vi "TEST-SAOMM-Externaloffset.vi"(0 "Hexapod VRN":refnum<visa-resource-name>="COM4", 1 "Active Refnum":refnum<vi>, 2 "PrAMS-ACK":refnum<vi>, 7 "output cluster":T2, 12 "offset_cluster":T1, 13 "MessageType":cluster{string[], u32[]}={["emtError", "emtAreYouThere", "emtAcknowledgment", "emtGetClientType", "emtClientType", "emtGetImageExposureTime", "emtSetImageExposureTime", "emtImageExposureTime", "emtGetOptimalExposureTime", "emtSetOptimalExposureTime", "emtOptimalExposureTime", "emtGetImageEMGain", "emtSetImageEMGain", "emtImageEMGain", "emtGetFPGACtrl", "emtSetFPGACtrl", "emtFPGACtrl", "emtGetImageWidth", "emtSetImageWidth", "emtImageWidth", "emtGetImageHeight", "emtSetImageHeight", "emtImageHeight", "emtGetImageBinning", "emtSetImageBinning", "emtImageBinning", "emtGetImageDisplayFrameRate", "emtSetImageDisplayFrameRate", "emtImageDisplayFrameRate", "emtGetROIWidth", "emtSetROIWidth", "emtROIWidth", "emtGetROIHeight", "emtSetROIHeight", "emtROIHeight", "emtGetROIXOffset", "emtSetROIXOffset", "emtROIXOffset", "emtGetROIYOffset", "emtSetROIYOffset", "emtROIYOffset", "emtStartAcquisition", "mtStopAcquisition", "emtAcquisitionStarted", "emtAcquisitionStopped", "emtGetFalconImage", "emtFalconImage"], [1, 2, 3, 4, 5, 1001, 1101, 1201, 1002, 1102, 1202, 1003, 1103, 1203, 1004, 1104, 1204, 1005, 1105, 1205, 1006, 1106, 1206, 1007, 1107, 1207, 1008, 1108, 1208, 1009, 1109, 1209, 1010, 1110, 1210, 1011, 1111, 1211, 1012, 1112, 1212, 1130, 1131, 1150, 1151, 1070, 1270]}) -> (8 "Error":bool)   [LabVIEW 2019]
uses:
  Polymorphics/Num2littleEndian(DBL).vi
panel:
  out "First Run":bool
  in  "IncUV":dbl caption="Incrément" format="%.4g"
  in  "IncXYZ":dbl caption="Incrément" format="%.3f"
  in  "V+":bool
  in  "V-":bool
  in  "U+":bool
  in  "U-":bool
  in  "Z+":bool
  in  "Z-":bool
  in  "Y+":bool
  in  "Y-":bool
  in  "X+":bool
  in  "X-":bool
  in  "keep-active":bool caption="Laisser ouvert ?"
  in  "Signature":u32=1886544237
  in  "Cancel":bool
  in  "Send":bool
  in  "X":dbl caption="Pos" min=-5.0 max=5.0 format="%.4f"
  in  "Y":dbl caption="Pos" min=-5.0 max=5.0 format="%.4f"
  in  "Z":dbl caption="Pos" min=-5.0 max=5.0 format="%.4f"
  in  "U":dbl caption="Pos" min=-1.0 max=1.0 format="%.4f"
  in  "V":dbl caption="Pos" min=-1.0 max=1.0 format="%.4f"
  # "DÉPLACEMENTS"
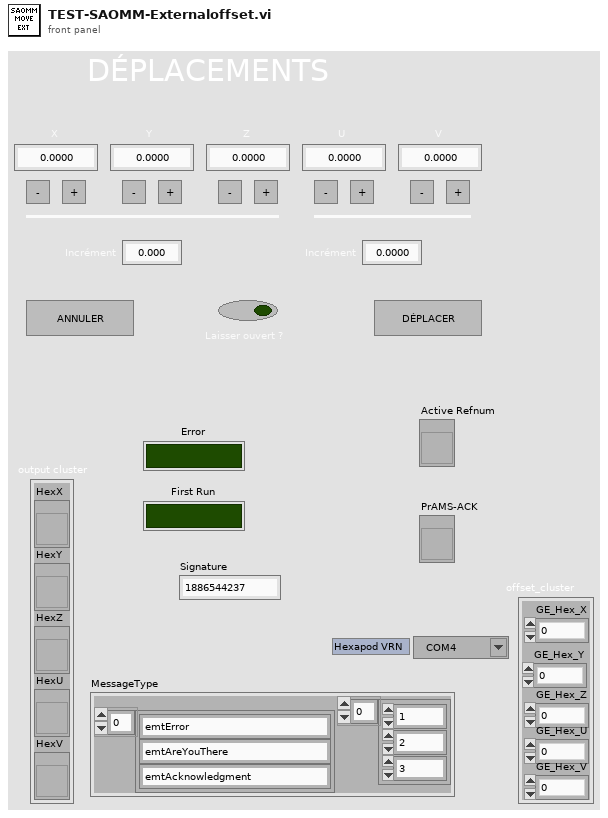
[diagram p1: front panel]
types:
  T1 = cluster{"GE_Hex_X":dbl, "GE_Hex_Y":dbl, "GE_Hex_Z":dbl, "GE_Hex_U":dbl, "GE_Hex_V":dbl}
  T2 = cluster{"HexX":refnum<vi>, "HexY":refnum<vi>, "HexZ":refnum<vi>, "HexU":refnum<vi>, "HexV":refnum<vi>}
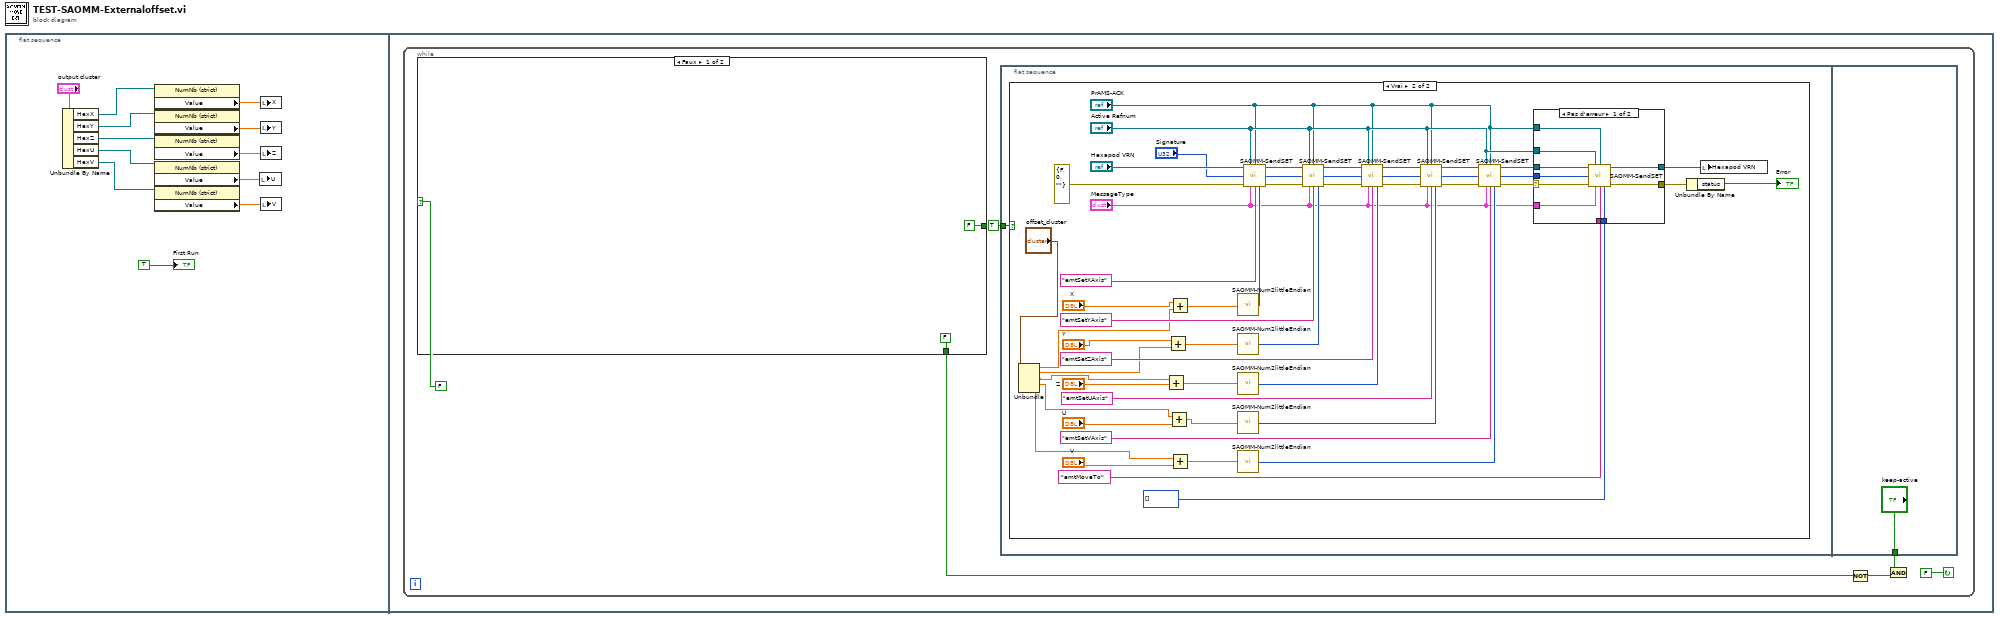
[diagram p0: block diagram]
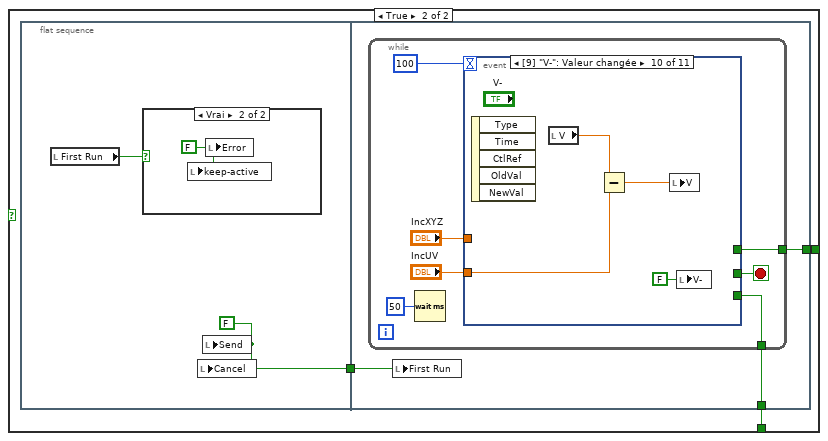
[diagram p2: hidden frame]
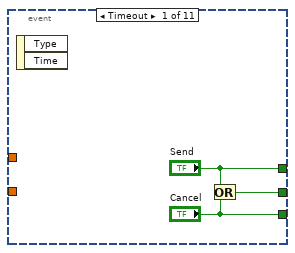
[diagram p4: hidden frame]
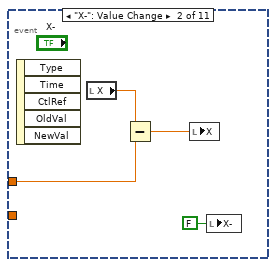
[diagram p5: hidden frame]
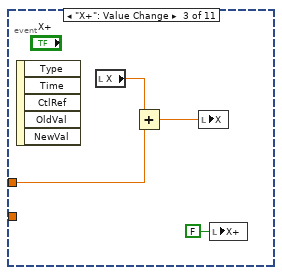
[diagram p6: hidden frame]
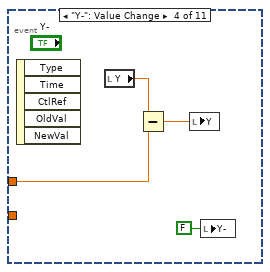
[diagram p7: hidden frame]
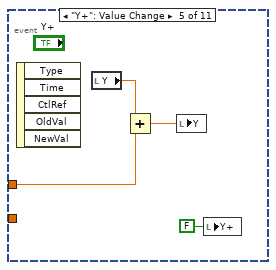
[diagram p8: hidden frame]
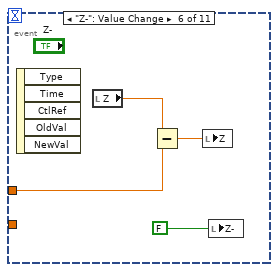
[diagram p9: hidden frame]
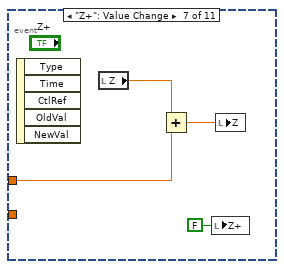
[diagram p10: hidden frame]
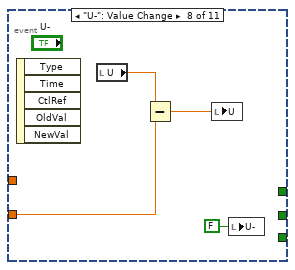
[diagram p11: hidden frame]
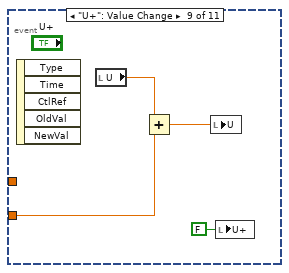
[diagram p12: hidden frame]
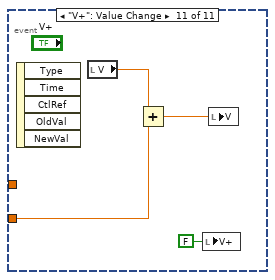
[diagram p13: hidden frame]
diagram:
  n1 = flat-sequence {
    frame #0 {
      n2 = Unbundle By Name("output cluster") -> ("HexX"=w10:refnum<vi>, "HexY"=w9:refnum<vi>, "HexZ"=w8:refnum<vi>, "HexU"=w7:refnum<vi>, "HexV"=w6:refnum<vi>)
      n3 = property class="NumNb (strict)"(reference=w10) -> ("Value"=w1:dbl)  [unwired: 1 in, 2 out]
      n4 = property class="NumNb (strict)"(reference=w9) -> ("Value"=w2:dbl)  [unwired: 1 in, 2 out]
      n5 = property class="NumNb (strict)"(reference=w8) -> ("Value"=w3:dbl)  [unwired: 1 in, 2 out]
      n6 = property class="NumNb (strict)"(reference=w7) -> ("Value"=w4:dbl)  [unwired: 1 in, 2 out]
      n7 = property class="NumNb (strict)"(reference=w6) -> ("Value"=w5:dbl)  [unwired: 1 in, 2 out]
      n8 = local write "U"(w4) -> ()
      n9 = local write "X"(w1) -> ()
      n10 = local write "Y"(w2) -> ()
      n11 = local write "Z"(w3) -> ()
      n12 = local write "V"(w5) -> ()
      "First Run" <- TRUE
    }
    frame #1 {
      n13 = while {
        stop <- FALSE continue-if-true
        n14 = case shown="Faux" FALSE {
          tunnel: [FALSE ("Send") w22] -> _
          tunnel: [FALSE ("Cancel") w21] -> w16
          frame False {
          }
          frame True {
            n15 = flat-sequence {
              tunnel: [w25] -> w23
              tunnel: [w28] -> w21
              tunnel: [w29] -> w22
              tunnel: w23 -> [w27]
              frame #0 {
                w25 = FALSE
                n16 = local read "First Run"() -> (w24:bool)
                n17 = case shown="Vrai" w24 {
                  frame False {
                  }
                  frame True {
                    w26 = FALSE ("Error")
                    n18 = local write "keep-active"(w26) -> ()
                    n19 = local write "Error"(w26) -> ()
                  }
                }
                n20 = local write "Cancel"(w25) -> ()
                n21 = local write "Send"(w25) -> ()
              }
              frame #1 {
                n22 = while {
                  tunnel: [w33] -> w29
                  tunnel: [w32] -> w28
                  stop <- w34 stop-if-true
                  n23 = Wait (ms)(milliseconds to wait=u32 50) -> ()  [unwired: 1 out]
                  n24 = event shown="[9] \"V-\": Valeur changée" {
                    selector: _ -> [_ _ _ _ _ _ _ _ _ _ _]
                    dyn-events: _ -> [_ _ _ _ _ _ _ _ _ _ _]
                    timeout: 100 -> [_ _ _ _ _ _ _ _ _ _ _]
                    tunnel: [w39 _ _ _ _ _ _ _ _ _ _] -> w34
                    tunnel: ["Send" _ _ _ _ _ _ _ _ _ _] -> w33
                    tunnel: ["Cancel" _ _ _ _ _ _ _ _ _ _] -> w32
                    tunnel: "IncXYZ" -> [_ w43 w45 w49 w53 w59 w61 _ _ _ _]
                    tunnel: "IncUV" -> [_ _ _ _ _ _ _ w65 w69 w74 w77]
                    event Timeout {
                      n25 = event-data() -> ()  [unwired: 1 in, 2 out]
                      n26 = Or(x="Send", y="Cancel") -> (x .or. y?=w39:bool)
                    }
                    event "X-": Value Change {
                      n27 = event-data() -> ()  [unwired: 1 in, 5 out]
                      n28 = local read "X"() -> (w41:dbl)
                      n29 = Subtract(x=w41, y=w43) -> (x-y=w42:dbl)
                      n30 = local write "X"(w42) -> ()
                      n31 = local write "X-"(FALSE ("X-")) -> ()
                    }
                    event "X+": Value Change {
                      n32 = event-data() -> ()  [unwired: 1 in, 5 out]
                      n33 = local read "X"() -> (w46:dbl)
                      n34 = Add(x=w46, y=w45) -> (x+y=w47:dbl)
                      n35 = local write "X"(w47) -> ()
                      n36 = local write "X+"(FALSE ("X+")) -> ()
                    }
                    event "Y-": Value Change {
                      n37 = event-data() -> ()  [unwired: 1 in, 5 out]
                      n38 = local read "Y"() -> (w51:dbl)
                      n39 = Subtract(x=w51, y=w49) -> (x-y=w50:dbl)
                      n40 = local write "Y"(w50) -> ()
                      n41 = local write "Y-"(FALSE ("Y-")) -> ()
                    }
                    event "Y+": Value Change {
                      n42 = event-data() -> ()  [unwired: 1 in, 5 out]
                      n43 = local read "Y"() -> (w55:dbl)
                      n44 = Add(x=w55, y=w53) -> (x+y=w54:dbl)
                      n45 = local write "Y"(w54) -> ()
                      n46 = local write "Y+"(FALSE ("Y+")) -> ()
                    }
                    event "Z-": Value Change {
                      n47 = event-data() -> ()  [unwired: 1 in, 5 out]
                      n48 = local read "Z"() -> (w58:dbl)
                      n49 = Subtract(x=w58, y=w59) -> (x-y=w57:dbl)
                      n50 = local write "Z"(w57) -> ()
                      n51 = local write "Z-"(FALSE ("Z-")) -> ()
                    }
                    event "Z+": Value Change {
                      n52 = event-data() -> ()  [unwired: 1 in, 5 out]
                      n53 = local read "Z"() -> (w63:dbl)
                      n54 = Add(x=w63, y=w61) -> (x+y=w62:dbl)
                      n55 = local write "Z+"(FALSE ("Z+")) -> ()
                      n56 = local write "Z"(w62) -> ()
                    }
                    event "U-": Value Change {
                      n57 = event-data() -> ()  [unwired: 1 in, 5 out]
                      n58 = local read "U"() -> (w67:dbl)
                      n59 = Subtract(x=w67, y=w65) -> (x-y=w66:dbl)
                      n60 = local write "U"(w66) -> ()
                      n61 = local write "U-"(FALSE ("U-")) -> ()
                    }
                    event "U+": Value Change {
                      n62 = event-data() -> ()  [unwired: 1 in, 5 out]
                      n63 = local read "U"() -> (w71:dbl)
                      n64 = Add(x=w71, y=w69) -> (x+y=w70:dbl)
                      n65 = local write "U"(w70) -> ()
                      n66 = local write "U+"(FALSE ("U+")) -> ()
                    }
                    event "V-": Value Change {
                      n67 = event-data() -> ()  [unwired: 1 in, 5 out]
                      n68 = local read "V"() -> (w75:dbl)
                      n69 = Subtract(x=w75, y=w74) -> (x-y=w73:dbl)
                      n70 = local write "V"(w73) -> ()
                      n71 = local write "V-"(FALSE ("V-")) -> ()
                    }
                    event "V+": Value Change {
                      n72 = event-data() -> ()  [unwired: 1 in, 5 out]
                      n73 = local read "V"() -> (w79:dbl)
                      n74 = Add(x=w79, y=w77) -> (x+y=w78:dbl)
                      n75 = local write "V+"(FALSE ("V+")) -> ()
                      n76 = local write "V"(w78) -> ()
                    }
                  }
                }
                n77 = local write "First Run"(w27) -> ()
              }
            }
          }
        }
        n78 = flat-sequence {
          tunnel: TRUE ("Send") -> [w80]
          tunnel: ["keep-active"] -> w18
          frame #0 {
            n79 = case shown="Vrai" w80 {
              frame False {
              }
              frame True {
                n80 = Unbundle("offset_cluster") -> ("GE_Hex_X"=w93:dbl, "GE_Hex_Y"=w90:dbl, "GE_Hex_Z"=w87:dbl, "GE_Hex_U"=w86:dbl, "GE_Hex_V"=w81:dbl)
                n81 = Add(x=w87, y="Z") -> (x+y=w88:dbl)
                n82 = Add(x="Y", y=w90) -> (x+y=w91:dbl)
                n83 = Add(x=w86, y="U") -> (x+y=w84:dbl)
                n84 = Add(x="X", y=w93) -> (x+y=w95:dbl)
                n85 = Add(x=w81, y="V") -> (x+y=w83:dbl)
                n86 = call-poly "SAOMM-Num2littleEndian.vi"("Number"=w95) -> ("LiitleEndianedData"=w114:u8[])  [unwired: 14 in]
                n87 = call-poly "SAOMM-Num2littleEndian.vi"("Number"=w91) -> ("LiitleEndianedData"=w115:u8[])  [unwired: 14 in]
                n88 = call-poly "SAOMM-Num2littleEndian.vi"("Number"=w88) -> ("LiitleEndianedData"=w116:u8[])  [unwired: 14 in]
                n89 = call-poly "SAOMM-Num2littleEndian.vi"("Number"=w84) -> ("LiitleEndianedData"=w119:u8[])  [unwired: 14 in]
                n90 = call-poly "SAOMM-Num2littleEndian.vi"("Number"=w83) -> ("LiitleEndianedData"=w120:u8[])  [unwired: 14 in]
                n91 = call "SAOMM-SendSET.vi"("PRAMMS-COMM IN"="Hexapod VRN", "Active Refnum"="Active Refnum", "PrAMS-ACK"="PrAMS-ACK", "Signature"="Signature", "Error IN"=errorcluster {"status"=FALSE, "code"=0, "source"=""}, "MessageType"="MessageType", "Active SET"="emtSetXAxis", "Value (little endianed byte array)"=w114) -> ("PRAMMS-COMM OUT"=w105:refnum<visa-resource-name>, "Error OUT"=w111:errorcluster)  [unwired: 4 in, 2 out]
                n92 = call "SAOMM-SendSET.vi"("PRAMMS-COMM IN"=w105, "Active Refnum"="Active Refnum", "PrAMS-ACK"="PrAMS-ACK", "Signature"="Signature", "Error IN"=w111, "MessageType"="MessageType", "Active SET"="emtSetYAxis", "Value (little endianed byte array)"=w115) -> ("PRAMMS-COMM OUT"=w106:refnum<visa-resource-name>, "Error OUT"=w110:errorcluster)  [unwired: 4 in, 2 out]
                n93 = call "SAOMM-SendSET.vi"("PRAMMS-COMM IN"=w106, "Active Refnum"="Active Refnum", "PrAMS-ACK"="PrAMS-ACK", "Signature"="Signature", "Error IN"=w110, "MessageType"="MessageType", "Active SET"="emtSetZAxis", "Value (little endianed byte array)"=w116) -> ("PRAMMS-COMM OUT"=w126:refnum<visa-resource-name>, "Error OUT"=w109:errorcluster)  [unwired: 4 in, 2 out]
                n94 = call "SAOMM-SendSET.vi"("PRAMMS-COMM IN"=w126, "Active Refnum"="Active Refnum", "PrAMS-ACK"="PrAMS-ACK", "Signature"="Signature", "Error IN"=w109, "MessageType"="MessageType", "Active SET"="emtSetUAxis", "Value (little endianed byte array)"=w119) -> ("PRAMMS-COMM OUT"=w127:refnum<visa-resource-name>, "Error OUT"=w108:errorcluster)  [unwired: 4 in, 2 out]
                n95 = call "SAOMM-SendSET.vi"("PRAMMS-COMM IN"=w127, "Active Refnum"="Active Refnum", "PrAMS-ACK"="PrAMS-ACK", "Signature"="Signature", "Error IN"=w108, "MessageType"="MessageType", "Active SET"="emtSetVAxis", "Value (little endianed byte array)"=w120) -> ("PRAMMS-COMM OUT"=w125:refnum<visa-resource-name>, "Error OUT"=w124:errorcluster)  [unwired: 4 in, 2 out]
                n96 = case shown="Pas d'erreur" w124 {
                  selector: w124 -> [w129 w138]
                  tunnel: "Active Refnum" -> [w137 _]
                  tunnel: "PrAMS-ACK" -> [w136 _]
                  tunnel: "Signature" -> [w135 _]
                  tunnel: [w134 w139] -> w107
                  tunnel: [w133 w138] -> w98
                  tunnel: "MessageType" -> [w132 _]
                  tunnel: "emtMoveTo" -> [w131 _]
                  tunnel: u8[] [] ("Value (little endianed byte array)") -> [w130 _]
                  tunnel: w125 -> [w128 w139]
                  frame No Error {
                    n97 = call "SAOMM-SendSET.vi"("PRAMMS-COMM IN"=w128, "Active Refnum"=w137, "PrAMS-ACK"=w136, "Signature"=w135, "Error IN"=w129, "MessageType"=w132, "Active SET"=w131, "Value (little endianed byte array)"=w130) -> ("PRAMMS-COMM OUT"=w134:refnum<visa-resource-name>, "Error OUT"=w133:errorcluster)  [unwired: 4 in, 2 out]
                  }
                  frame Error {
                  }
                }
                n98 = Unbundle By Name(w98) -> ("status"=→"Error":bool)
                n99 = local write "Hexapod VRN"(w107) -> ()
              }
            }
          }
          frame #1 {
          }
        }
        n100 = Not(x=w16) -> (.not. x?=w17:bool)
        n101 = And(x=w18, y=w17) -> ()  [unwired: 1 out]
      }
    }
  }
